vi "_PC_Pub_Var2Type.vi"(3 "Input Variable":variant) -> (0 "Output Name":string[](array[string]), 1 "Output Type":T1[](array[typedef]) format="%.0x")   [LabVIEW 2018]
uses:
  <userlib>/_OpenG.lib/lvdata/lvdata.llb/Type Descriptor Enumeration__ogtk.ctl
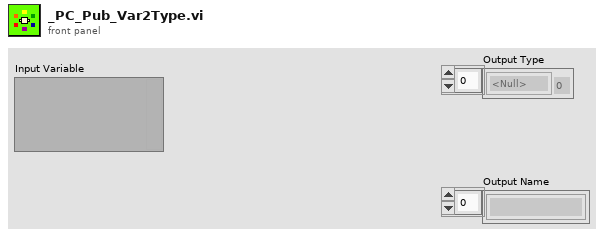
[diagram p1: front panel]
types:
  T1 = typedef "Type Descriptor Enumeration__ogtk.ctl" = enum8{"<Null>", "I8", "I16", "I32", "I64", "U8", "U16", "U32", "U64", "SGL", "DBL", "EXT", "CSG", "CDB", "CXT", "0x0F", "0x10", "0x11", "0x12", "0x13", "0x14", "Enum U8", "Enum U16", "Enum U32", "Enum U64", "SGL PQ", "DBL PQ", "EXT PQ", "CSG PQ", "CDB PQ", "CXT PQ", "0x1F", "0x20", "Boolean", "0x22", "0x23", "0x24", "0x25", "0x26", "0x27", "0x28", "0x29", "0x2A", "0x2B", "0x2C", "0x2D", "0x2E", "0x2F", "String", "0x31", "Path", "Pict", "0x34", "0x35", "0x36", "DAQ", "0x38", "0x39", "0x3A", "0x3B", "0x3C", "0x3D", "0x3E", "0x3F", "Array", "0x41", "0x42", "0x43", "0x44", "0x45", "0x46", "0x47", "0x48", "0x49", "0x4A", "0x4B", "0x4C", "0x4D", "0x4E", "0x4F", "Cluster", "0x51", "0x52", "Variant", "Waveform", "0x55", "0x56", "0x57", "0x58", "0x59", "0x5A", "0x5B", "0x5C", "0x5D", "0x5E", "0x5F", "0x60", "0x61", "0x62", "0x63", "0x64", "0x65", "0x66", "0x67", "0x68", "0x69", "0x6A", "0x6B", "0x6C", "0x6D", "0x6E", "0x6F", "Refnum"}
  T2 = typedef "Type Descriptor__ogtk.ctl" = i16[]
  T3 = typedef "Type Descriptor Header__ogtk.ctl" = cluster{"length":u16, "private":u8, "type":T1, "# elements":u16}
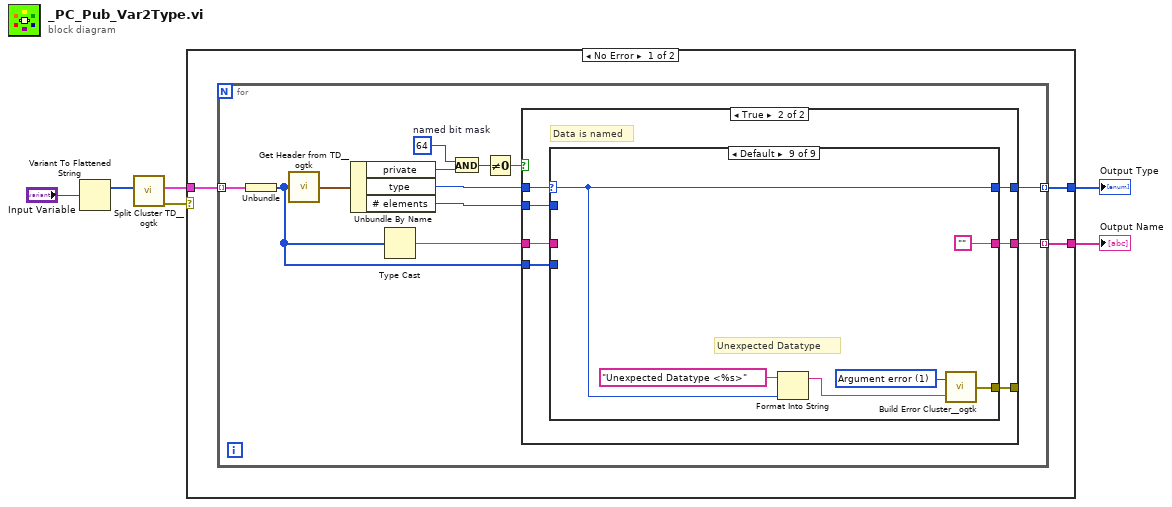
[diagram p0: block diagram]
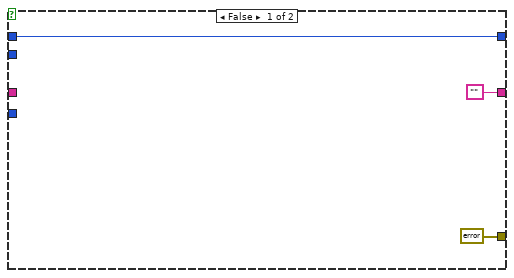
[diagram p2: hidden frame]
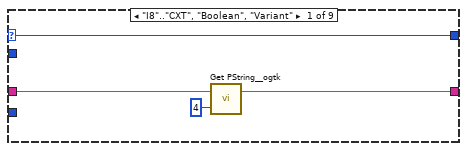
[diagram p3: hidden frame]
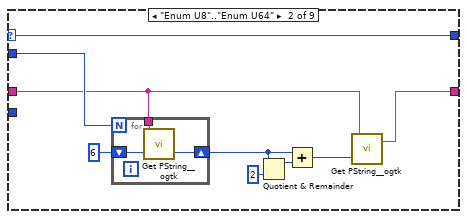
[diagram p4: hidden frame]
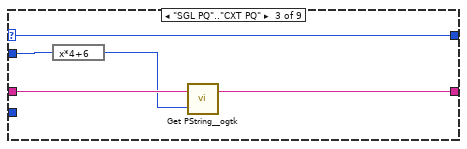
[diagram p5: hidden frame]
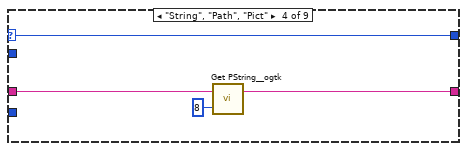
[diagram p6: hidden frame]
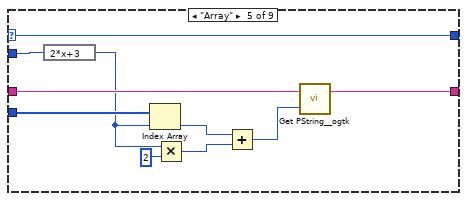
[diagram p7: hidden frame]
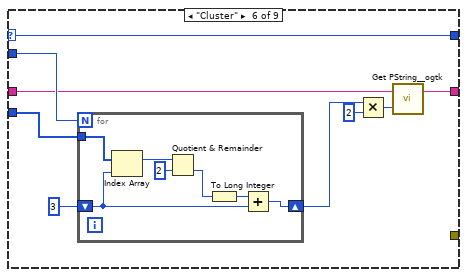
[diagram p8: hidden frame]
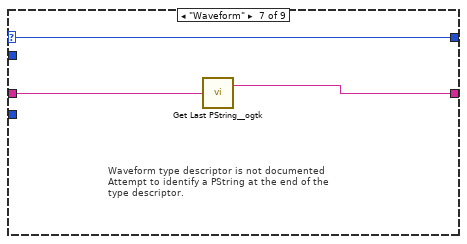
[diagram p9: hidden frame]
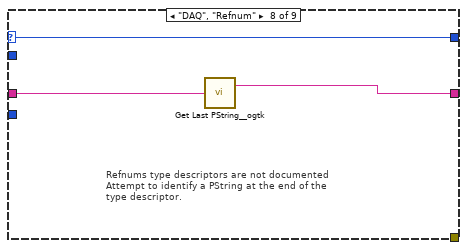
[diagram p10: hidden frame]
diagram:
  n1 = Variant To Flattened String(Variant="Input Variable") -> (1:w6:i16[])  [unwired: 1 out]
  n2 = call <userlib>:"Split Cluster TD__ogtk.vi"("Type Descriptor"=w6) -> ("error out"=w1:errorcluster, "Type Descriptors"=w5:cluster{"Type Descriptor":T2}[])  [unwired: 9 in]
  n3 = case shown="No Error" w1 {
    tunnel: w5 -> [w9 _]
    tunnel: [w8 _] -> w4
    tunnel: [w7 _] -> w2
    frame No Error {
      n4 = for {
        tunnel: w9 -> [w21] mode=indexing
        tunnel: [w11] -> w8 mode=indexing
        tunnel: [w10] -> w7 mode=indexing
        w19 = u8 64  # named bit mask
        n5 = Unbundle(w21) -> ("Type Descriptor"=w14:T2)
        n6 = call <userlib>:"Get Header from TD__ogtk.vi"("Type Descriptor"=w14) -> ("Type Descriptor Header"=w20:T3)
        n7 = Unbundle By Name(w20) -> ("private"=w18:u8, "type"=w17:T1, "# elements"=w16:u16)
        n8 = Type Cast(x=w14) -> (*(type *) &x=w15:string)  [unwired: 1 in]
        n9 = And(x=w19, y=w18) -> (x .and. y?=w13:u8)
        n10 = Not Equal To 0?(x=w13) -> (x != 0?=w12:bool)
        n11 = case shown="True" w12 {
          tunnel: [errorcluster {"status"=FALSE, "code"=0, "source"=""} ("error out") w31] -> _
          tunnel: w17 -> [w22 w30]
          tunnel: w15 -> [_ w29]
          tunnel: ["" w28] -> w11
          tunnel: w16 -> [_ w27]
          tunnel: w14 -> [_ w26]
          tunnel: [w22 w25] -> w10
          frame False {
          }
          frame True {
            # "Data is named"
            n12 = case shown="Default" w30 {
              selector: w30 -> [w32 w36 w48 w53 w57 w67 w83 w86 w89]
              tunnel: [_ _ _ _ _ _ _ _ w94] -> w31
              tunnel: w29 -> [w35 w37 w51 w56 w64 w73 w85 w88 _]
              tunnel: [w33 w41 w49 w55 w60 w72 w84 w87 ""] -> w28
              tunnel: w27 -> [_ w40 w52 _ w66 w75 _ _ _]
              tunnel: w26 -> [_ _ _ _ w65 w74 _ _ _]
              tunnel: [w32 w36 w48 w53 w57 w67 w83 w86 w89] -> w25
              frame "I8".."CXT", "Boolean", "Variant" {
                n13 = call <userlib>:"Get PString__ogtk.vi"("offset (0)"=4, "String"=w35) -> ("PString"=w33:string)  [unwired: 1 out]
              }
              frame "Enum U8".."Enum U64" {
                n14 = for {
                  N: w40 -> [_]
                  tunnel: w37 -> [w45]
                  shift-right: [w46] -> w43
                  shift-left: 6 -> [w47]
                  n15 = call <userlib>:"Get PString__ogtk.vi"("offset (0)"=w47, "String"=w45) -> ("offset past PString"=w46:i32)  [unwired: 1 out]
                }
                n16 = Quotient & Remainder(x=w43, y=2) -> (x-y*floor(x/y)=w38:i32)  [unwired: 1 out]
                n17 = Add(x=w43, y=w38) -> (x+y=w42:i32)
                n18 = call <userlib>:"Get PString__ogtk.vi"("offset (0)"=w42, "String"=w37) -> ("PString"=w41:string)  [unwired: 1 out]
              }
              frame "SGL PQ".."CXT PQ" {
                n19 = expression code="x*4+6"(w52) -> (w50:u16)
                n20 = call <userlib>:"Get PString__ogtk.vi"("offset (0)"=w50, "String"=w51) -> ("PString"=w49:string)  [unwired: 1 out]
              }
              frame "String", "Path", "Pict" {
                n21 = call <userlib>:"Get PString__ogtk.vi"("offset (0)"=8, "String"=w56) -> ("PString"=w55:string)  [unwired: 1 out]
              }
              frame "Array" {
                n22 = expression code="2*x+3"(w66) -> (w63:u16)
                n23 = Index Array(array=w65, index=w63) -> (element=w58:i16)
                n24 = Multiply(x=w63, y=u16 2) -> (x*y=w59:u16)
                n25 = Add(x=w58, y=w59) -> (x+y=w61:u16)
                n26 = call <userlib>:"Get PString__ogtk.vi"("offset (0)"=w61, "String"=w64) -> ("PString"=w60:string)  [unwired: 1 out]
              }
              frame "Cluster" {
                n27 = for {
                  N: w75 -> [_]
                  shift-right: [w81] -> w70
                  shift-left: 3 -> [w80]
                  tunnel: w74 -> [w82]
                  n28 = Index Array(array=w82, index=w80) -> (element=w78:i16)
                  n29 = Quotient & Remainder(x=w78, y=i16 2) -> (floor(x/y)=w79:i16)  [unwired: 1 out]
                  n30 = To Long Integer(number=w79) -> (32bit integer=w76:i32)
                  n31 = Add(x=w76, y=w80) -> (x+y=w81:i32)
                }
                n32 = Multiply(x=w70, y=2) -> (x*y=w69:i32)
                n33 = call <userlib>:"Get PString__ogtk.vi"("offset (0)"=w69, "String"=w73) -> ("PString"=w72:string)  [unwired: 1 out]
              }
              frame "Waveform" {
                # "Waveform type descriptor is not documented\nAttempt to identify a PString at the end of the\ntype descriptor."
                n34 = call <userlib>:"Get Last PString__ogtk.vi"("String"=w85) -> ("Last PString"=w84:string)  [unwired: 1 out]
              }
              frame "DAQ", "Refnum" {
                # "Refnums type descriptors are not documented\nAttempt to identify a PString at the end of the\ntype descriptor."
                n35 = call <userlib>:"Get Last PString__ogtk.vi"("String"=w88) -> ("Last PString"=w87:string)  [unwired: 1 out]
              }
              frame Default {
                w93 = 1 items=["No error", "Argument error", "Memory is full", "Out of zone", "End of file", "File already open", "Generic file I/O error", "File not found", "File permission error", "Disk is full", "Duplicate path", "Too many files open", "System feature not enabled", "Resource file not found", "Cannot add resource", "Resource not found", "Image not found", "Image memory error", "Pen does not exist", "Config type invalid", "Config token not found", "Config parse error", "Config memory error", "Bad external code format", "Bad external code offset", "External code not present", "Null window", "Destroy window error", "Null menu", "Print aborted", "Bad print record", "Print driver error", "Windows error during printing", "Memory error during printing", "Print dialog error", "Generic print error", "Invalid device refnum", "Device not found", "Device parameter error", "Device unit error", "Cannot open device", "Device call aborted", "Generic error", "Cancelled by user", "Object ID too low", "Object ID too high", "Object not in heap", "Unknown heap", "Unknown object (invalid DefProc)", "Unknown object (DefProc not in table)", "Message out of range", "Invalid (null) method", "Unknown message", "Manager call not supported", "Bad address", "Network operation in progress", "Network operation timed out", "Connection is busy", "Network attribute not supported", "Network error", "Address in use", "System out of memory", "Connection aborted", "Connection refused", "Not connected", "Already connected", "Connection closed", "Initialization error (interapplication manager)", "Bad occurrence", "Wait on unbound occurrence handler", "Occurrence queue overflow", "Datalog type conflict", "Unused", "Unrecognized type (interapplication manager)", "Memory corrupt", "Failed to make temporary DLL", "Old CIN version", "Drag socket not found", "Failed to load drop-object", "Failed to register OLE object", "Failed to release OLE object", "Format specifier type mismatch", "Unknown format specifier", "Too few format specifiers", "Too many format specifiers", "Scan failed", "Newer CIN version", "Error converting to variant", "Runtime menu error", "Password tampered", "Variant attribute not found", "Incompatible variant data type", "Event data is not available", "Event Store is not present", "Occurrence is not found", "Event Queue is not created", "Event info is not available", "Refnum passed is NULL", "Error retrieving Class GUID", "Error retrieving CoClass GUID", "Error retrieving TypeLib GUID.", "Bad built application magic bytes.", "Specific driver is different from the specific driver associated with the Logical Name.", "There is no session opened to the class driver.", "Max Error", "MAX - Error with config objects", "MAX - Error loading configuration", "MAX - Group not supported"]
                # "Unexpected Datatype"
                n36 = Format Into String(format string="Unexpected Datatype <%s>" ("Format String"), w89) -> (resulting string=w90:string)  [unwired: 2 in, 1 out]
                n37 = call <userlib>:"Build Error Cluster__ogtk.vi"("String to Prepend to source (\"\")"=w90, "code"=w93) -> ("error out"=w94:errorcluster)
              }
            }
          }
        }
      }
    }
    frame Error {
    }
  }
  "Output Name" <- w4
  "Output Type" <- w2
